vi "TEST_L1_COMPLETE_ALL.vi"() -> ()   [LabVIEW 2012]
uses:
  <vilib>/Utility/NIReport.llb/NI_report.lvclass
  <vilib>/Utility/NIReport.llb/HTML/NI_HTML.lvclass
panel:
  in  "Initialisation Check":bool=TRUE
  in  "Baseline":bool=TRUE
  in  "Adder Test":bool=TRUE
  in  "Transfer Function":bool=TRUE
  in  "Instrument VISA in":T1={"AWG VISA"="AgilentGen1", "Oscilloscope  VISA "="AgilentOsc", "Integration Board IP"="172.16.17.48", "connection ID"=refnum, "report out"=refnum, "report file path"=path "C:/Users/omartinez/Desktop/L0nL1_Results"}
  out "Instrument VISA out":T1={"AWG VISA"="AgilentGen1", "Oscilloscope  VISA "="AgilentOsc", "Integration Board IP"="172.16.17.48", "connection ID"=refnum, "report out"=refnum, "report file path"=path "C:/Users/omartinez/Desktop/L0nL1_Results"}
  out "error out":errorcluster {"code" format="%f"}
  in  "error in":errorcluster
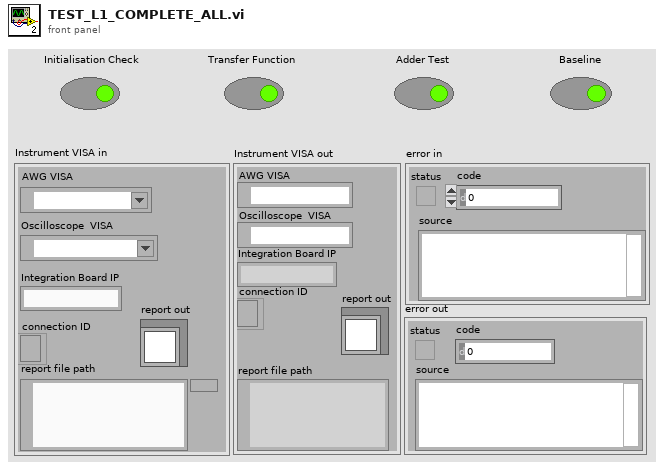
[diagram p1: front panel]
types:
  T1 = cluster{"AWG VISA":refnum<visa-resource-name>, "Oscilloscope  VISA ":refnum<visa-resource-name>, "Integration Board IP":string, "connection ID":refnum<k5>, "report out":refnum<class "NI_report.lvclass">, "report file path":path}
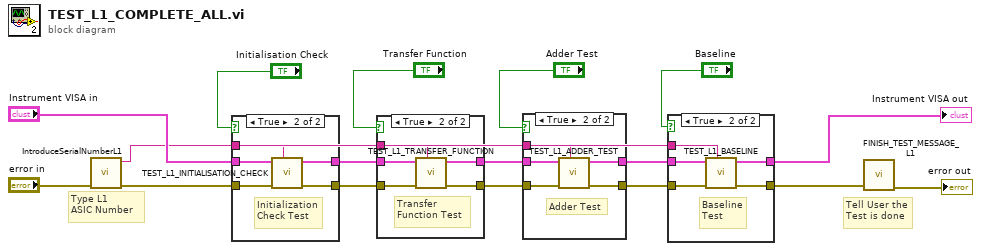
[diagram p0: block diagram]
diagram:
  # "Tell User the\nTest is done"
  # "Type L1\nASIC Number"
  n1 = call "IntroduceSerialNumberL1.vi"("error in"="error in") -> ("error out"=w3:errorcluster, "Serial Number"=w1:string)  [unwired: 9 in]
  n2 = case shown="True" "Initialisation Check" {
    tunnel: [w19 w20] -> w5
    tunnel: [w18 w21] -> w4
    tunnel: "Instrument VISA in" -> [w19 w24]
    tunnel: w3 -> [w18 w22]
    tunnel: w1 -> [_ w23]
    frame False {
    }
    frame True {
      # "Initialization\nCheck Test"
      n3 = call "TEST_L1_INITIALISATION_CHECK.vi"("Serial Number"=w23, "error in"=w22, "VISA IN"=w24) -> ("error out"=w21:errorcluster, "VISA OUT"=w20:T1)  [unwired: 5 in]
    }
  }
  n4 = case shown="True" "Transfer Function" {
    tunnel: [w26 w31] -> w17
    tunnel: [w25 w30] -> w14
    tunnel: w5 -> [w26 w28]
    tunnel: w4 -> [w25 w29]
    tunnel: w1 -> [_ w27]
    frame False {
    }
    frame True {
      # "Transfer\nFunction Test"
      n5 = call "TEST_L1_TRANSFER_FUNCTION.vi"("Serial Number"=w27, "error in"=w29, "Instrument VISA in"=w28) -> ("error out"=w30:errorcluster, "VISA Out"=w31:T1)  [unwired: 5 in]
    }
  }
  n6 = case shown="True" "Adder Test" {
    tunnel: w17 -> [w33 w37]
    tunnel: [w33 w36] -> w16
    tunnel: w14 -> [w32 w35]
    tunnel: [w32 w38] -> w13
    tunnel: w1 -> [_ w34]
    frame False {
    }
    frame True {
      # "Adder Test"
      n7 = call "TEST_L1_ADDER_TEST.vi"("Serial Number"=w34, "error in"=w35, "Instrument VISA in"=w37) -> ("error out"=w38:errorcluster, "VISA Out"=w36:T1)  [unwired: 5 in]
    }
  }
  n8 = case shown="True" "Baseline" {
    tunnel: w16 -> [w40 w43]
    tunnel: [w40 w42] -> w15
    tunnel: w13 -> [w39 w44]
    tunnel: [w39 w45] -> w7
    tunnel: w1 -> [_ w41]
    frame False {
    }
    frame True {
      # "Baseline\nTest"
      n9 = call "TEST_L1_BASELINE.vi"("Serial Number"=w41, "error in"=w44, "Instrument VISA in"=w43) -> ("error out"=w45:errorcluster, "VISA Out"=w42:T1)  [unwired: 5 in]
    }
  }
  "Instrument VISA out" <- w15
  n10 = call "FINISH_TEST_MESSAGE_L1.vi"("error in"=w7) -> ("error out"=→"error out":errorcluster)  [unwired: 10 in]
